vi "Generate Random GB of Size 2014-11-13.vi"() -> ()   [LabVIEW 2010]
uses:
  <vilib>/Utility/file.llb/Write To Spreadsheet File (string).vi
panel:
  out "# Created":i32
  out "Grain Boundary Definition":T1={"Grain 1 Orientation"=[1.0, 0.8858401549498205, 0.0], "Grain 2 Orientation"=[1.0, 0.3745791306245927, 0.0], "Twist Angle (Deg)"=39.42112887005932, "Translation Vector"=[0.0, 0.0, 0.0]}
  out "Current Index":i32=165102
  out "Status":string="Within range!\nNow creating...\nChecking expected size\nRolling dice...\n"
  in  "Make Random GBs Tab":T2(tab)=enum."Constraints"
  in  "Random Space":enum32{"Interface Plane", "Misorientation"}(tab)
  in  "Grain 1 Orientation":T3={"h, minimum"=1.0, "h, maximum"=1.0, "k, minimum"=0.0, "k, maximum"=1.0, "l, minimum"=0.0, "l, maximum"=1.0, "Force h>k>l ?"=TRUE} {"h, minimum" format="%#_4f"; "h, maximum" format="%#_4f"; "k, minimum" format="%#_4f"; "k, maximum" format="%#_4f"; "l, minimum" format="%#_4f"; "l, maximum" format="%#_4f"}
  in  "Random Translation?":bool
  in  "Twist Angle Max":dbl=64.0
  in  "Twist Angle Min":dbl
  in  "Grain 2 Orientation":T3={"h, minimum"=1.0, "h, maximum"=1.0, "k, minimum"=0.0, "k, maximum"=1.0, "l, minimum"=0.0, "l, maximum"=1.0, "Force h>k>l ?"=TRUE} {"h, minimum" format="%#_4f"; "h, maximum" format="%#_4f"; "k, minimum" format="%#_4f"; "k, maximum" format="%#_4f"; "l, minimum" format="%#_4f"; "l, maximum" format="%#_4f"}
  in  "Random Translation? Mis":bool
  in  "Mis Angle Max":dbl=64.0
  in  "Mis Angle Min":dbl
  in  "Misorientation Axis":T3={"h, minimum"=1.0, "h, maximum"=1.0, "k, minimum"=0.0, "k, maximum"=1.0, "l, minimum"=0.0, "l, maximum"=1.0, "Force h>k>l ?"=TRUE} {"h, minimum" format="%#_4f"; "h, maximum" format="%#_4f"; "k, minimum" format="%#_4f"; "k, maximum" format="%#_4f"; "l, minimum" format="%#_4f"; "l, maximum" format="%#_4f"}
  in  "Interface Plane from Grain 1":T3={"h, minimum"=1.0, "h, maximum"=1.0, "k, minimum"=0.0, "k, maximum"=1.0, "l, minimum"=0.0, "l, maximum"=1.0, "Force h>k>l ?"=TRUE} {"h, minimum" format="%#_4f"; "h, maximum" format="%#_4f"; "k, minimum" format="%#_4f"; "k, maximum" format="%#_4f"; "l, minimum" format="%#_4f"; "l, maximum" format="%#_4f"}
  in  "Nearest Integers?":bool
  in  "Max # of Atoms":i32=500
  in  "Require STEM Viewable?":bool
  in  "Grain Growth and Geometry":T4={"Grain 1 Length (prop)"=10.0, "Grain 2 Length (prop)"=10.0, "Max Grain Height (A)"=60.0, "Max Grain Width (A)"=60.0, "Grain 1 Start"=-0.001, "Overlap Region (A)"=0.001}
  in  "Min Seperation Distance (A)":dbl=2.0
  in  "Edge Duplication Range":dbl=3.0
  out "Expected # of atoms":i32=472
  out "# of atoms":i32=2541
  in  "Reduce to Repeating":T5={"Slab X"=4.6, "Slab Y"=4.0, "Tolerance (A)"=0.5, "Presorted?"=FALSE}
  in  "Output Directory":path=path "D:/Ab-initio/RAGB3"
  out "Last Creation Time":T6={"Time to create primitives"=1, "Time to Grow to Box"=5932, "Time to find subset"=6894, "Time to Cleanup"=0}
  out "Structures / Minute":dbl
  in  "Stop Making GBs":bool
  in  "Start Making GBs":bool
  in  "Making GBs":bool=TRUE
  in  "Conventional Unit Cell":T7={"Structure Name"="CdTe", "Lattice vector a"=[6.615785553057252, 0.0, 0.0], "Lattice vector b"=[0.0, 6.615785553057252, 0.0], "Lattice vector c"=[0.0, 0.0, 6.615785553057252], "Atoms Array"=[{"Atom Name"="Cd", "Positions (Direct)"=[[0.0, 0.0, 0.0], [0.0, 0.5, 0.5], [0.5, 0.0, 0.5], [0.5, 0.5, 0.0]], "Positions (Cartesian)"=[[0.0, 0.0, 0.0], [0.0, 3.307892776528626, 3.307892776528626], [3.307892776528626, 0.0, 3.307892776528626], [3.307892776528626, 3.307892776528626, 0.0]]}, {"Atom Name"="Te", "Positions (Direct)"=[[0.25, 0.25, 0.25], [0.75, 0.75, 0.25], [0.75, 0.25, 0.75], [0.25, 0.75, 0.75]], "Positions (Cartesian)"=[[1.653946388264313, 1.653946388264313, 1.653946388264313], [4.96183916479294, 4.96183916479294, 1.653946388264313], [4.96183916479294, 1.653946388264313, 4.96183916479294], [1.653946388264313, 4.96183916479294, 4.96183916479294]]}], "# of atoms"=8}
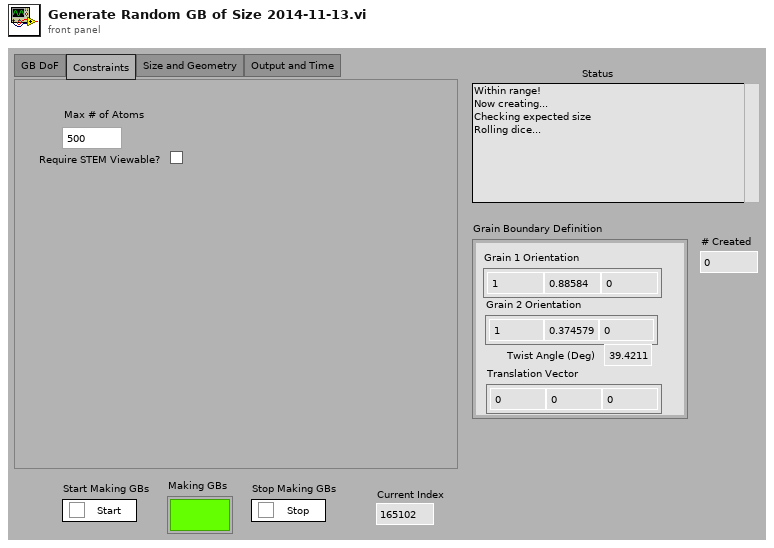
[diagram p1: front panel]
types:
  T1 = cluster{"Grain 1 Orientation":dbl[], "Grain 2 Orientation":dbl[], "Twist Angle (Deg)":dbl, "Translation Vector":dbl[]}
  T2 = enum32{"GB DoF", "Constraints", "Size and Geometry", "Output and Time"}
  T3 = cluster{"h, minimum":dbl, "h, maximum":dbl, "k, minimum":dbl, "k, maximum":dbl, "l, minimum":dbl, "l, maximum":dbl, "Force h>k>l ?":bool}
  T4 = cluster{"Grain 1 Length (prop)":dbl, "Grain 2 Length (prop)":dbl, "Max Grain Height (A)":dbl, "Max Grain Width (A)":dbl, "Grain 1 Start":dbl, "Overlap Region (A)":dbl}
  T5 = cluster{"Slab X":dbl, "Slab Y":dbl, "Tolerance (A)":dbl, "Presorted?":bool}
  T6 = cluster{"Time to create primitives":u32, "Time to Grow to Box":u32, "Time to find subset":u32, "Time to Cleanup":u32}
  T7 = cluster{"Structure Name":string, "Lattice vector a":dbl[], "Lattice vector b":dbl[], "Lattice vector c":dbl[], "Atoms Array":cluster{"Atom Name":string, "Positions (Direct)":dbl[][], "Positions (Cartesian)":dbl[][]}[], "# of atoms":i32}
  T8 = cluster{"Grain 1 Orientation":dbl[], "Grain 1 Orientation":dbl[], "Twist Angle (Deg)":dbl, "Translation Vector":dbl[]}
  T9 = cluster{"Grain 1 Orientation":dbl[], "Grain 2 Orientation":dbl[], "Twist Angle (Deg)":dbl}
  T10 = cluster{"Structure Name":string, "Lattice vector a":dbl[], "Lattice vector b":dbl[], "Lattice vector c":dbl[], "Atoms Array":cluster{"Atom Name":string, "Positions (Direct)":dbl[][], "Positions (Cartesian)":dbl[][]}[], "# of atoms":i32}[]
  T11 = typedef "NI_Matrix.lvlib/RealMatrix.ctl" = dbl[][]
  T12 = cluster{"Misorientation Angle":dbl, "Misorientation Axis, o":dbl[], "Misorientation Matrix":T11}
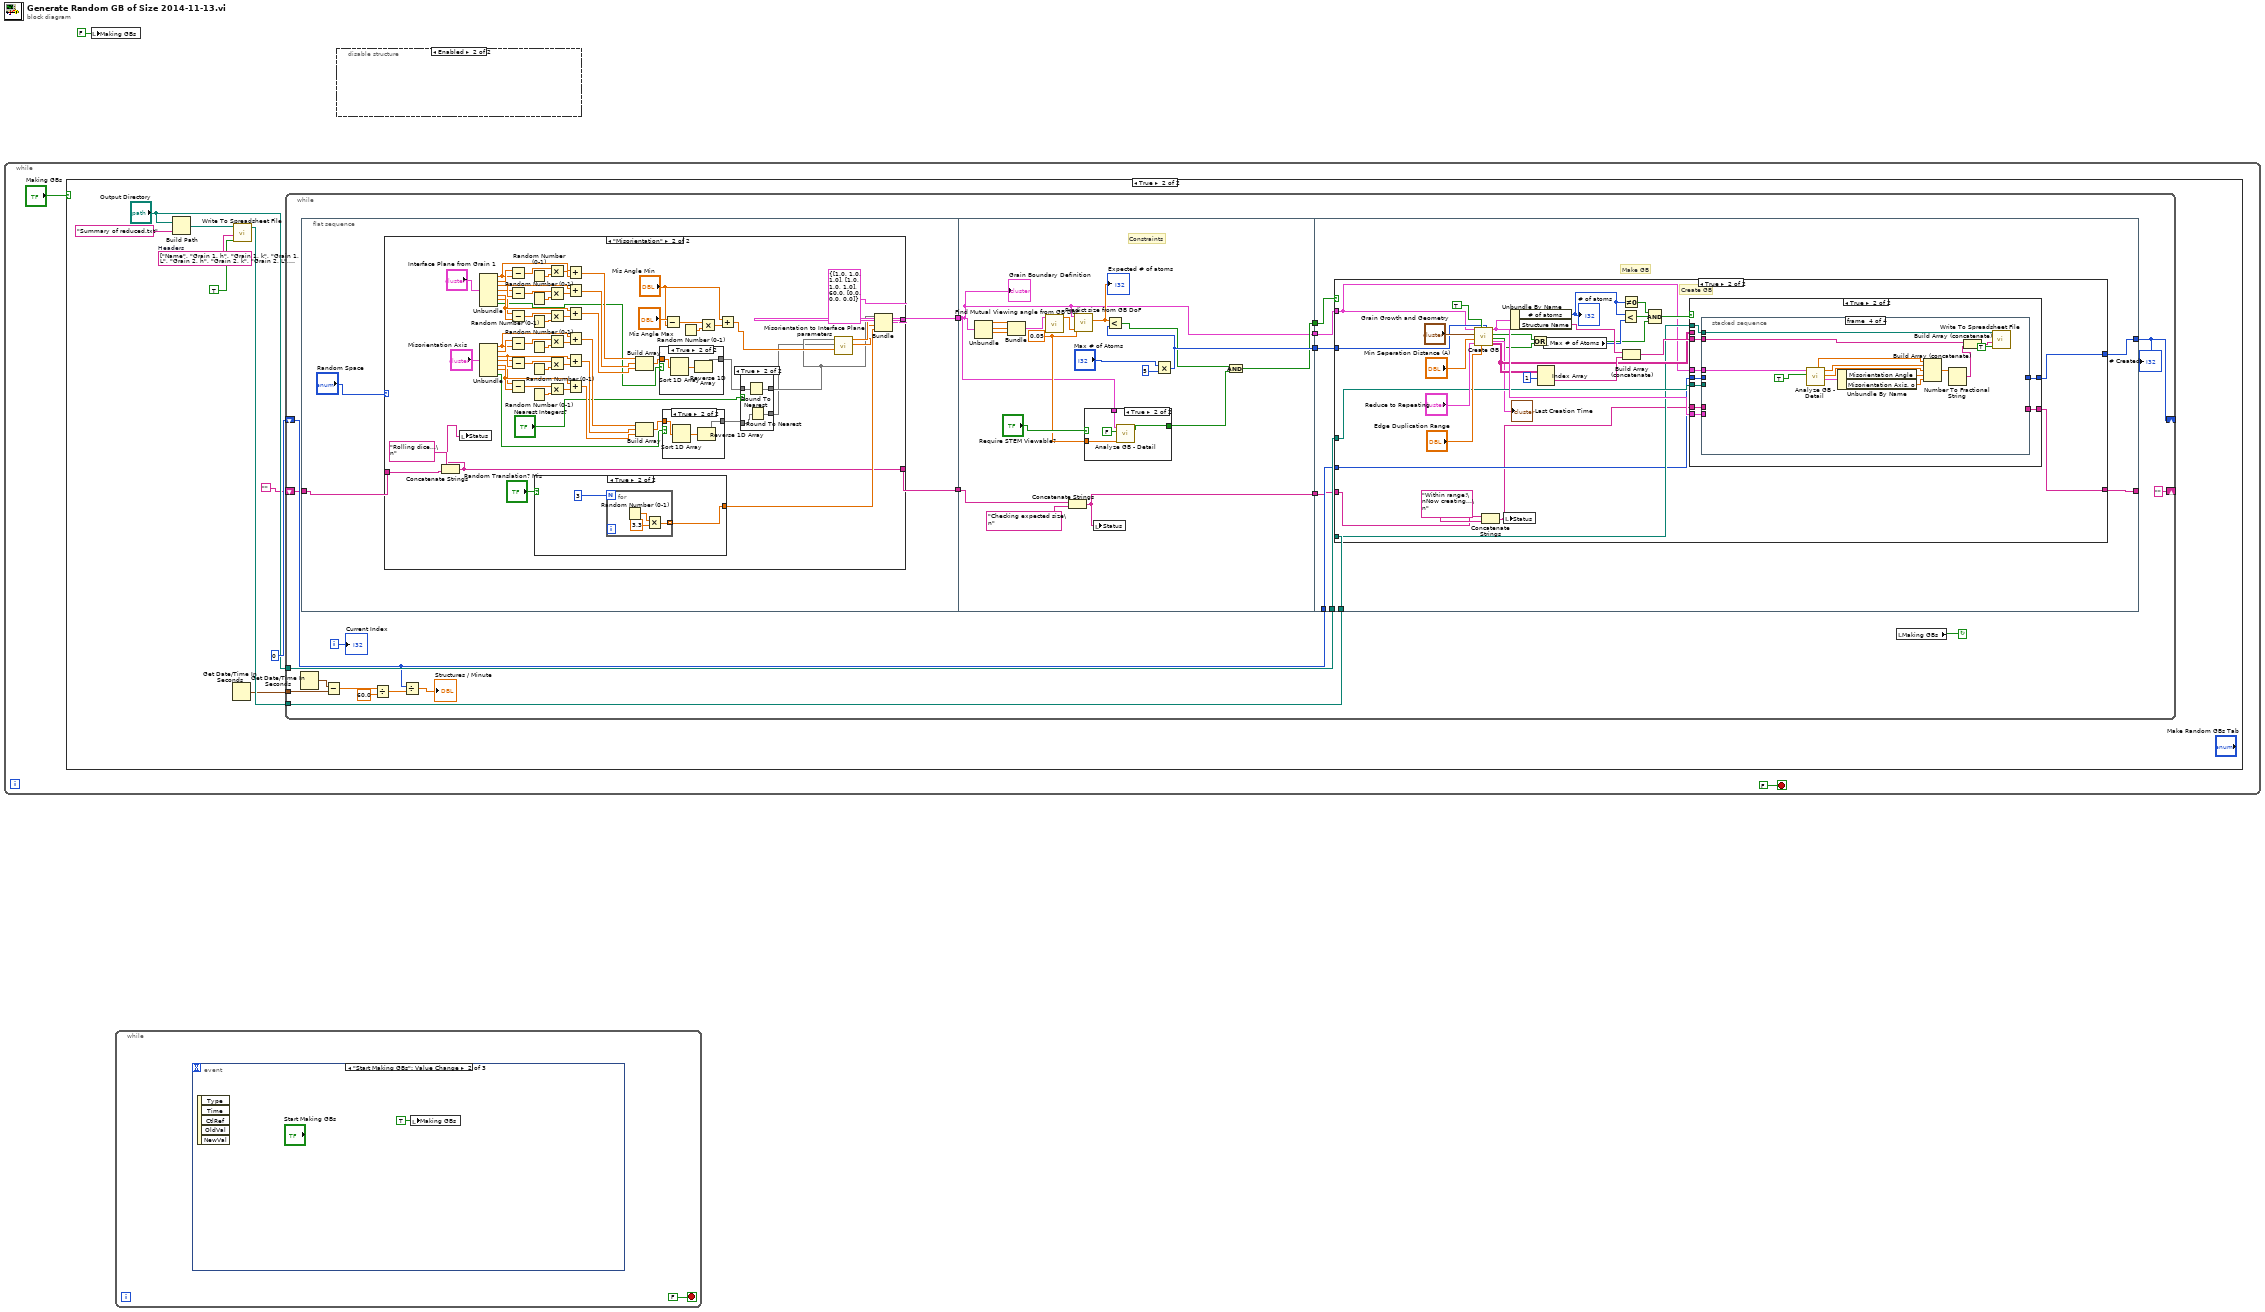
[diagram p0: block diagram]
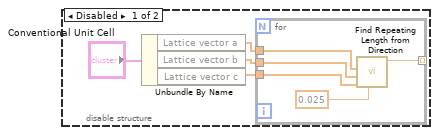
[diagram p2: hidden frame]
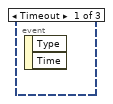
[diagram p3: hidden frame]
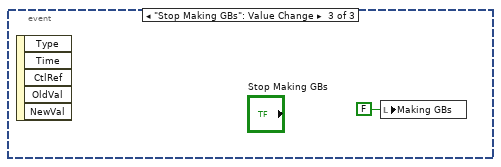
[diagram p4: hidden frame]
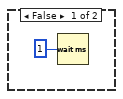
[diagram p5: hidden frame]
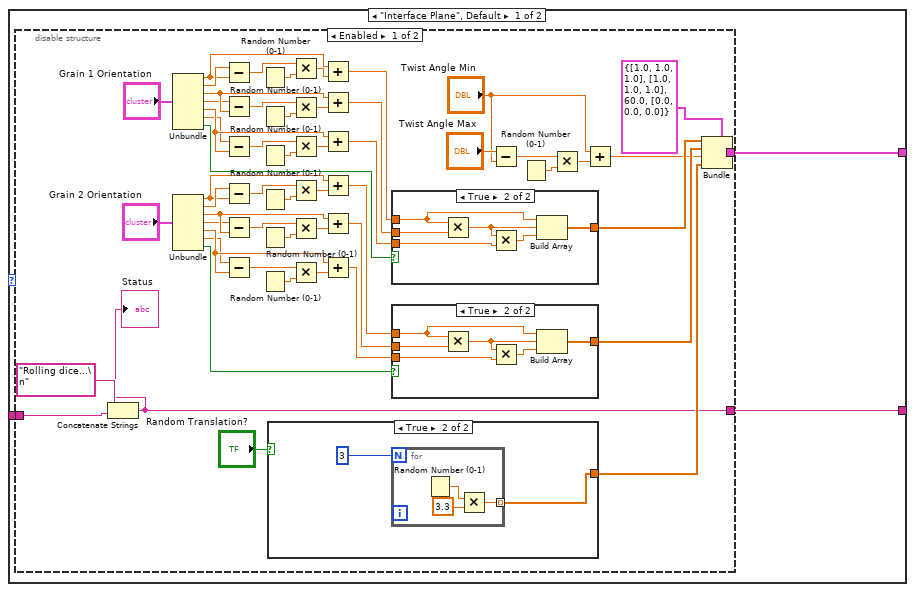
[diagram p6: hidden frame]
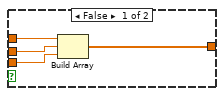
[diagram p7: hidden frame]
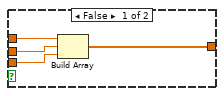
[diagram p8: hidden frame]
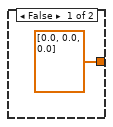
[diagram p9: hidden frame]
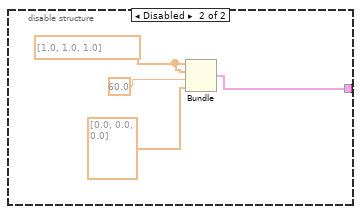
[diagram p10: hidden frame]
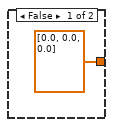
[diagram p14: hidden frame]
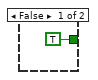
[diagram p15: hidden frame]
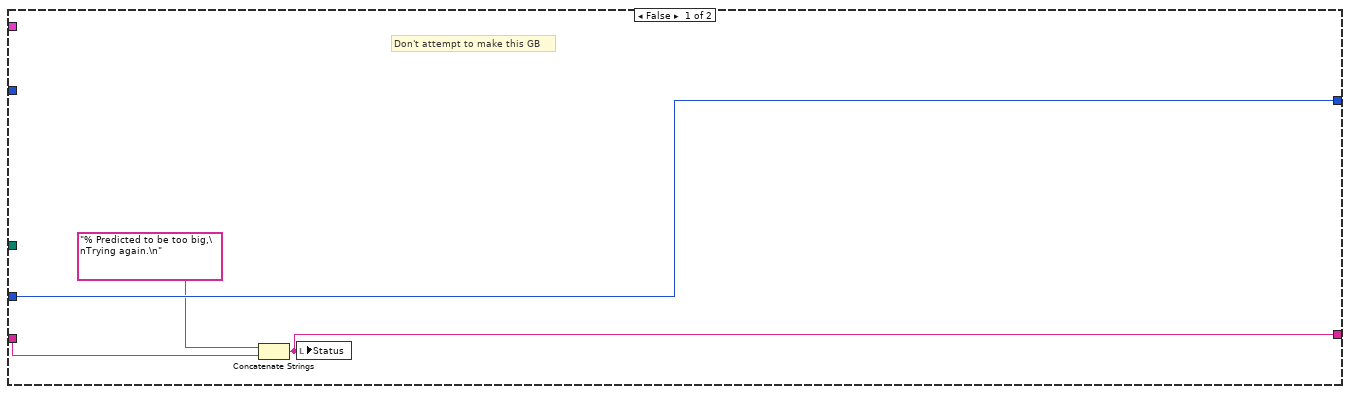
[diagram p16: hidden frame]
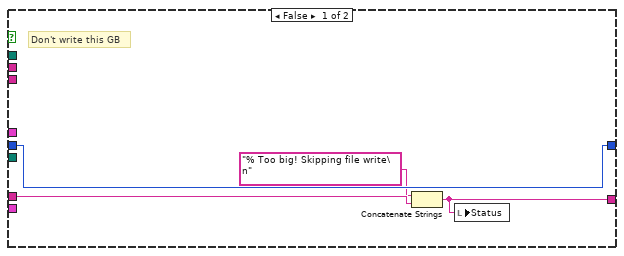
[diagram p17: hidden frame]
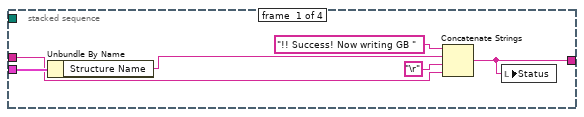
[diagram p18: hidden frame]
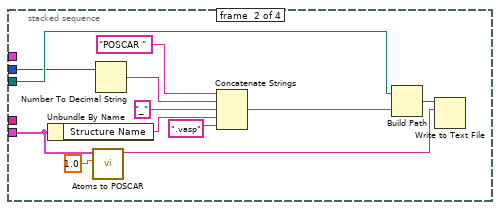
[diagram p19: hidden frame]
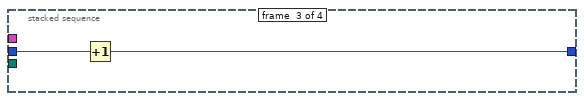
[diagram p20: hidden frame]
diagram:
  n1 = while {
    stop <- FALSE stop-if-true
    n2 = case shown="True" "Making GBs" {
      frame False {
        n3 = Wait (ms)(milliseconds to wait=u32 1) -> ()  [unwired: 1 out]
      }
      frame True {
        w9 = string[] ["Name", "Grain 1, h", "Grain 1, k", "Grain 1, L", "Grain 2, h", "Grain 2, k", "Grain 2, L", "Twist Angle (Deg)", "Translation Tx", "Translation Ty", "Translation Tz", "Tilt Angle (Deg)", "Viewing Angle, h", "Viewing Angle, k", "Viewing Angle, L", "Grain 1 Length (factor)", "Grain 2 Length (factor", "Max Grain Height (A)", "Max Grain Width (A)", "Grain 1 Start", "Overlap Region (A)", "Reduction Slab X", "Reduction Slab Y", "Reduction Tolerance (A)", "Min Atomic Separation Distance", "Edge Duplication Range", "# of Atoms", "STEM Direction,h", "STEM Direction,k", "STEM Direction,l", "Grain 1, [h]", "Grain 1, [k]", "Grain 1, [L]", "Grain 2, [h]", "Grain 2, [k]", "Grain 2, [L]", "Misorientaton Angle (Deg)", "Misorientation Axis, h", "Misorientation Axis, k", "Misorientation Axis, l"]  # Headers
        n4 = Build Path(base path="Output Directory", name or relative path="Summary of reduced.txt") -> (appended path=w10:path)
        n5 = Get Date/Time In Seconds() -> (seconds since 1Jan1904=w5:timestamp)
        n6 = call-poly <vilib>:"Write To Spreadsheet File.vi"("append to file? (new file:F)"=TRUE, "1D data"=w9, "file path (dialog if empty)"=w10) -> ("new file path (Not A Path if cancelled)"=w7:path)  [unwired: 5 in]
        n7 = while {
          shift-right: [w21] -> _
          shift-left: 0 -> [w22]
          tunnel: w5 -> [w29]
          tunnel: "Output Directory" -> [w24]
          tunnel: w7 -> [w23]
          shift-right: [""] -> _
          shift-left: "" -> [w20]
          i -> [w33]
          stop <- w17 continue-if-true
          n8 = Get Date/Time In Seconds() -> (seconds since 1Jan1904=w14:timestamp)
          n9 = flat-sequence {
            tunnel: [w37] -> w27
            tunnel: w20 -> [w36]
            tunnel: [w35] -> w19
            tunnel: w27 -> [w212]
            tunnel: [w212] -> w26
            tunnel: [w214] -> w25
            tunnel: w19 -> [w223]
            tunnel: [w221] -> w18
            tunnel: [w218] -> w15
            tunnel: w26 -> [w235]
            tunnel: w25 -> [w239]
            tunnel: w24 -> [w238]
            tunnel: w23 -> [w237]
            tunnel: w22 -> [w236]
            tunnel: [w234] -> w21
            tunnel: w18 -> [w233]
            tunnel: [w232] -> _
            tunnel: w15 -> [w231]
            frame #0 {
              n10 = case shown="\"Misorientation\"" "Random Space" {
                tunnel: [w40 w187] -> w37
                tunnel: w36 -> [w39 w140]
                tunnel: [w38 w135] -> w35
                frame "Interface Plane", Default {
                  n11 = disable-structure shown="Enabled" {
                    disable-tunnel: [w95 w122] -> w40
                    disable-tunnel: w39 -> [w43 _]
                    disable-tunnel: [w41 _] -> w38
                    frame Enabled {
                      n12 = Concatenate Strings(w43, "Rolling dice...\n" ("string")) -> (w41:string)
                      "Status" <- w41
                      n13 = Unbundle("Grain 1 Orientation") -> ("h, minimum"=w88:dbl, "h, maximum"=w91:dbl, "k, minimum"=w83:dbl, "k, maximum"=w82:dbl, "l, minimum"=w81:dbl, "l, maximum"=w80:dbl, "Force h>k>l ?"=w79:bool)
                      n14 = Unbundle("Grain 2 Orientation") -> ("h, minimum"=w68:dbl, "h, maximum"=w71:dbl, "k, minimum"=w63:dbl, "k, maximum"=w62:dbl, "l, minimum"=w61:dbl, "l, maximum"=w60:dbl, "Force h>k>l ?"=w59:bool)
                      n15 = Subtract(x=w91, y=w88) -> (x-y=w90:dbl)
                      n16 = Subtract(x=w82, y=w83) -> (x-y=w86:dbl)
                      n17 = Subtract(x=w80, y=w81) -> (x-y=w85:dbl)
                      n18 = Subtract(x=w71, y=w68) -> (x-y=w70:dbl)
                      n19 = Subtract(x=w62, y=w63) -> (x-y=w66:dbl)
                      n20 = Subtract(x=w60, y=w61) -> (x-y=w65:dbl)
                      n21 = Random Number (0-1)() -> (number: 0 to 1=w77:dbl)
                      n22 = Random Number (0-1)() -> (number: 0 to 1=w76:dbl)
                      n23 = Random Number (0-1)() -> (number: 0 to 1=w75:dbl)
                      n24 = Random Number (0-1)() -> (number: 0 to 1=w57:dbl)
                      n25 = Random Number (0-1)() -> (number: 0 to 1=w56:dbl)
                      n26 = Random Number (0-1)() -> (number: 0 to 1=w55:dbl)
                      n27 = case shown="True" "Random Translation?" {
                        tunnel: [dbl[] [0.0, 0.0, 0.0] w117] -> w94
                        frame False {
                        }
                        frame True {
                          n28 = for {
                            N: 3 -> [_]
                            tunnel: [w119] -> w117 mode=indexing
                            n29 = Random Number (0-1)() -> (number: 0 to 1=w121:dbl)
                            n30 = Multiply(x=w121, y=3.3) -> (x*y=w119:dbl)
                          }
                        }
                      }
                      n31 = Multiply(x=w90, y=w77) -> (x*y=w89:dbl)
                      n32 = Multiply(x=w86, y=w76) -> (x*y=w87:dbl)
                      n33 = Multiply(x=w85, y=w75) -> (x*y=w84:dbl)
                      n34 = Multiply(x=w70, y=w57) -> (x*y=w69:dbl)
                      n35 = Multiply(x=w66, y=w56) -> (x*y=w67:dbl)
                      n36 = Multiply(x=w65, y=w55) -> (x*y=w64:dbl)
                      n37 = Add(x=w88, y=w89) -> (x+y=w78:dbl)
                      n38 = Add(x=w83, y=w87) -> (x+y=w74:dbl)
                      n39 = Add(x=w81, y=w84) -> (x+y=w73:dbl)
                      n40 = Add(x=w68, y=w69) -> (x+y=w58:dbl)
                      n41 = Add(x=w63, y=w67) -> (x+y=w54:dbl)
                      n42 = Add(x=w61, y=w64) -> (x+y=w53:dbl)
                      n43 = case shown="True" w79 {
                        tunnel: w78 -> [w109 w113]
                        tunnel: w74 -> [w108 w115]
                        tunnel: w73 -> [w107 w114]
                        tunnel: [w106 w110] -> w72
                        frame False {
                          n44 = Build Array(w109, w108, w107) -> (w106:dbl[])
                        }
                        frame True {
                          n45 = Multiply(x=w113, y=w115) -> (x*y=w112:dbl)
                          n46 = Multiply(x=w112, y=w114) -> (x*y=w111:dbl)
                          n47 = Build Array(w113, w112, w111) -> (w110:dbl[])
                        }
                      }
                      n48 = case shown="True" w59 {
                        tunnel: w58 -> [w99 w103]
                        tunnel: w54 -> [w98 w105]
                        tunnel: w53 -> [w97 w104]
                        tunnel: [w96 w100] -> w52
                        frame False {
                          n49 = Build Array(w99, w98, w97) -> (w96:dbl[])
                        }
                        frame True {
                          n50 = Multiply(x=w103, y=w105) -> (x*y=w102:dbl)
                          n51 = Multiply(x=w102, y=w104) -> (x*y=w101:dbl)
                          n52 = Build Array(w103, w102, w101) -> (w100:dbl[])
                        }
                      }
                      n53 = Subtract(x="Twist Angle Max", y="Twist Angle Min") -> (x-y=w48:dbl)
                      n54 = Random Number (0-1)() -> (number: 0 to 1=w50:dbl)
                      n55 = Multiply(x=w48, y=w50) -> (x*y=w49:dbl)
                      n56 = Add(x="Twist Angle Min", y=w49) -> (x+y=w45:dbl)
                      n57 = Bundle(cluster=T1 {"Grain 1 Orientation"=[1.0, 1.0, 1.0], "Grain 2 Orientation"=[1.0, 1.0, 1.0], "Twist Angle (Deg)"=60.0, "Translation Vector"=[0.0, 0.0, 0.0]} ("Grain Boundary Definition"), "Grain 1 Orientation"=w72, "Grain 2 Orientation"=w52, "Twist Angle (Deg)"=w45, "Translation Vector"=w94) -> (w95:T1)
                    }
                    frame Disabled {
                      w125 = dbl[] [1.0, 1.0, 1.0] ("Grain 1 Orientation")
                      n58 = Bundle("Grain 1 Orientation"=w125, "Grain 1 Orientation"=w125, "Twist Angle (Deg)"=60.0, "Translation Vector"=dbl[] [0.0, 0.0, 0.0]) -> (w122:T8)  [unwired: 1 in]
                    }
                  }
                }
                frame "Misorientation" {
                  n59 = Concatenate Strings(w140, "Rolling dice...\n" ("string")) -> (w135:string)
                  n60 = local write "Status"(w135) -> ()
                  n61 = Unbundle("Interface Plane from Grain 1") -> ("h, minimum"=w180:dbl, "h, maximum"=w183:dbl, "k, minimum"=w175:dbl, "k, maximum"=w174:dbl, "l, minimum"=w173:dbl, "l, maximum"=w172:dbl, "Force h>k>l ?"=w129:bool)
                  n62 = Unbundle("Misorientation Axis") -> ("h, minimum"=w162:dbl, "h, maximum"=w165:dbl, "k, minimum"=w157:dbl, "k, maximum"=w156:dbl, "l, minimum"=w155:dbl, "l, maximum"=w154:dbl, "Force h>k>l ?"=w126:bool)
                  n63 = Subtract(x=w183, y=w180) -> (x-y=w182:dbl)
                  n64 = Subtract(x=w174, y=w175) -> (x-y=w178:dbl)
                  n65 = Subtract(x=w172, y=w173) -> (x-y=w177:dbl)
                  n66 = Subtract(x=w165, y=w162) -> (x-y=w164:dbl)
                  n67 = Subtract(x=w156, y=w157) -> (x-y=w160:dbl)
                  n68 = Subtract(x=w154, y=w155) -> (x-y=w159:dbl)
                  n69 = Random Number (0-1)() -> (number: 0 to 1=w170:dbl)
                  n70 = Random Number (0-1)() -> (number: 0 to 1=w169:dbl)
                  n71 = Random Number (0-1)() -> (number: 0 to 1=w168:dbl)
                  n72 = Random Number (0-1)() -> (number: 0 to 1=w152:dbl)
                  n73 = Random Number (0-1)() -> (number: 0 to 1=w151:dbl)
                  n74 = Random Number (0-1)() -> (number: 0 to 1=w150:dbl)
                  n75 = case shown="True" "Random Translation? Mis" {
                    tunnel: [dbl[] [0.0, 0.0, 0.0] w203] -> w186
                    frame False {
                    }
                    frame True {
                      n76 = for {
                        N: 3 -> [_]
                        tunnel: [w205] -> w203 mode=indexing
                        n77 = Random Number (0-1)() -> (number: 0 to 1=w207:dbl)
                        n78 = Multiply(x=w207, y=3.3) -> (x*y=w205:dbl)
                      }
                    }
                  }
                  n79 = Multiply(x=w182, y=w170) -> (x*y=w181:dbl)
                  n80 = Multiply(x=w178, y=w169) -> (x*y=w179:dbl)
                  n81 = Multiply(x=w177, y=w168) -> (x*y=w176:dbl)
                  n82 = Multiply(x=w164, y=w152) -> (x*y=w163:dbl)
                  n83 = Multiply(x=w160, y=w151) -> (x*y=w161:dbl)
                  n84 = Multiply(x=w159, y=w150) -> (x*y=w158:dbl)
                  n85 = Add(x=w180, y=w181) -> (x+y=w171:dbl)
                  n86 = Add(x=w175, y=w179) -> (x+y=w167:dbl)
                  n87 = Add(x=w173, y=w176) -> (x+y=w166:dbl)
                  n88 = Add(x=w162, y=w163) -> (x+y=w153:dbl)
                  n89 = Add(x=w157, y=w161) -> (x+y=w149:dbl)
                  n90 = Add(x=w155, y=w158) -> (x+y=w148:dbl)
                  n91 = Build Array(w171, w167, w166) -> (w130:dbl[])
                  n92 = Build Array(w153, w149, w148) -> (w128:dbl[])
                  n93 = case shown="True" w129 {
                    tunnel: [w192 w193] -> w131
                    tunnel: w130 -> [w192 w195]
                    frame False {
                    }
                    frame True {
                      n94 = Sort 1D Array(array=w195) -> (sorted array=w194:dbl[])
                      n95 = Reverse 1D Array(array=w194) -> (reversed array=w193:dbl[])
                    }
                  }
                  n96 = case shown="True" w126 {
                    tunnel: [w188 w189] -> w127
                    tunnel: w128 -> [w188 w190]
                    frame False {
                    }
                    frame True {
                      n97 = Sort 1D Array(array=w190) -> (sorted array=w191:dbl[])
                      n98 = Reverse 1D Array(array=w191) -> (reversed array=w189:dbl[])
                    }
                  }
                  n99 = Subtract(x="Mis Angle Max", y="Mis Angle Min") -> (x-y=w144:dbl)
                  n100 = Random Number (0-1)() -> (number: 0 to 1=w146:dbl)
                  n101 = Multiply(x=w144, y=w146) -> (x*y=w145:dbl)
                  n102 = Add(x="Mis Angle Min", y=w145) -> (x+y=w138:dbl)
                  n103 = case shown="True" "Nearest Integers?" {
                    tunnel: w127 -> [w196 w201]
                    tunnel: [w196 w200] -> w132
                    tunnel: w131 -> [w197 w199]
                    tunnel: [w197 w198] -> w133
                    frame False {
                    }
                    frame True {
                      n104 = Round To Nearest(number=w199) -> (nearest integer value=w198:dbl[])
                      n105 = Round To Nearest(number=w201) -> (nearest integer value=w200:dbl[])
                    }
                  }
                  n106 = call "Misorientation to Interface Plane parameters.vi"("Misorientation Angle"=w138, "Misorientation Axis, o"=w132, "Grain 1 Orientation"=w133) -> ("Twist Angle (Deg)"=w136:dbl, "Grain 2 Orientation"=w137:dbl[])  [unwired: 5 in, 2 out]
                  n107 = Bundle(cluster=T1 {"Grain 1 Orientation"=[1.0, 1.0, 1.0], "Grain 2 Orientation"=[1.0, 1.0, 1.0], "Twist Angle (Deg)"=60.0, "Translation Vector"=[0.0, 0.0, 0.0]} ("Grain Boundary Definition"), "Grain 1 Orientation"=w133, "Grain 2 Orientation"=w137, "Twist Angle (Deg)"=w136, "Translation Vector"=w186) -> (w187:T1)
                }
              }
            }
            frame #1 {
              w213 = 0.05 ("Integer Tolerance")
              # "Constraints"
              n108 = Unbundle(w212) -> ("Grain 1 Orientation"=w211:dbl[], "Grain 2 Orientation"=w210:dbl[], "Twist Angle (Deg)"=w209:dbl)  [unwired: 1 out]
              n109 = Bundle("Grain 1 Orientation"=w211, "Grain 2 Orientation"=w210, "Twist Angle (Deg)"=w209) -> (w208:T9)  [unwired: 1 in]
              n110 = call "Find Mutual Viewing angle from GB DoF.vi"("Grain Boundary Macro DoF"=w208) -> ("Mutual Viewing Angle"=w224:dbl[])  [unwired: 8 in, 2 out]
              n111 = Concatenate Strings(w223, "Checking expected size\n" ("string")) -> (w221:string)
              n112 = call "Predict size from GB DoF.vi"("Integer Tolerance"=w224, "Mutual Viewing Angle"=w213, "Grain Boundary Definition"=w212) -> ("Expected Volume (A3)"=w225:dbl)  [unwired: 6 in, 2 out]
              "Expected # of atoms" <- w225
              n113 = case shown="True" "Require STEM Viewable?" {
                tunnel: w212 -> [_ w229]
                tunnel: [TRUE ("STEM Viewable?") w228] -> w215
                tunnel: w213 -> [_ w227]
                frame False {
                }
                frame True {
                  n114 = call "Analyze GB - Detail.vi"("Integer Tolerance"=w227, "Find Integer Rep?"=FALSE, "Grain Boundary Definition"=w229) -> ("STEM Viewable?"=w228:bool)  [unwired: 1 in, 7 out]
                }
              }
              n115 = local write "Status"(w221) -> ()
              n116 = Multiply(x="Max # of Atoms", y=5) -> (x*y=w218:i32)
              n117 = Less?(x=w225, y=w218) -> (x < y?=w216:bool)
              n118 = And(x=w216, y=w215) -> (x .and. y?=w214:bool)
              "Grain Boundary Definition" <- w212
            }
            frame #2 {
              # "Make GB"
              n119 = case shown="True" w239 {
                tunnel: w238 -> [_ w263]
                tunnel: w237 -> [_ w262]
                tunnel: w236 -> [w243 w261]
                tunnel: w235 -> [_ w244]
                tunnel: [w243 w253] -> w234
                tunnel: w233 -> [w242 w251]
                tunnel: [w240 w249] -> w232
                tunnel: w231 -> [_ w245]
                frame False {
                  # "Don't attempt to make this GB"
                  n120 = Concatenate Strings("% Predicted to be too big,\nTrying again.\n" ("string"), w242) -> (w240:string)
                  n121 = local write "Status"(w240) -> ()
                }
                frame True {
                  # "Create GB"
                  n122 = call "Create GB.vi"("Max # of atoms"=w245, "Edge Duplication Range"="Edge Duplication Range", "Skip cleanup if no subset"=TRUE, "Reduce to Repeating"="Reduce to Repeating", "Min Seperation Distance (A)"="Min Seperation Distance (A)", "Grain Growth and Geometry"="Grain Growth and Geometry", "Grain Boundary Definition"=w244) -> ("GB Data"=w268:string[][], "Reduced Orthorhombic?"=w247:bool, "Reduced Rhombahedral?"=w248:bool, "Grain Boundary"=w269:T7, "Ortho and Rhom"=→"Last Creation Time":T10)
                  n123 = Concatenate Strings(w251, "Within range!\nNow creating...\n" ("string")) -> (w250:string)
                  n124 = local write "Status"(w250) -> ()
                  n125 = Unbundle By Name(w269) -> ("# of atoms"=w257:i32, "Structure Name"=w273:string)
                  "# of atoms" <- w257
                  n126 = Or(x=w248, y=w247) -> (x .or. y?=w246:bool)
                  n127 = Index Array(array=w268, index (row)=1) -> (element=w271:string[])  [unwired: 1 in]
                  n128 = local read "Max # of Atoms"() -> (w258:i32)
                  n129 = Less?(x=w257, y=w258) -> (x < y?=w255:bool)
                  n130 = Not Equal To 0?(x=w257) -> (x != 0?=w256:bool)
                  n131 = Build Array (concatenate)(w273, w271) -> (w272:string[])
                  n132 = Compound Arithmetic op=AND(w256, w255, w246) -> (w254:bool)
                  n133 = case shown="True" w254 {
                    tunnel: w261 -> [w277 w284]
                    tunnel: [w277 w283] -> w253
                    tunnel: w268 -> [_ _]
                    tunnel: w269 -> [_ w286]
                    tunnel: w272 -> [_ w281]
                    tunnel: w263 -> [_ w285]
                    tunnel: w262 -> [_ w282]
                    tunnel: w250 -> [w276 w279]
                    tunnel: [w275 w278] -> w249
                    tunnel: w244 -> [_ w280]
                    frame False {
                      # "Don't write this GB"
                      n134 = Concatenate Strings("% Too big! Skipping file write\n" ("string"), w276) -> (w275:string)
                      n135 = local write "Status"(w275) -> ()
                    }
                    frame True {
                      n136 = stacked-sequence {
                        tunnel: w286 -> [w290 w304 _ _]
                        tunnel: w285 -> [_ w299 _ _]
                        tunnel: w284 -> [_ w297 w306 _]
                        tunnel: [_ _ w305 _] -> w283
                        tunnel: w282 -> [_ _ _ w320]
                        tunnel: w281 -> [_ _ _ w318]
                        tunnel: w280 -> [_ _ _ w312]
                        tunnel: w279 -> [w288 _ _ _]
                        tunnel: [w287 _ _ _] -> w278
                        frame #0 {
                          n137 = Unbundle By Name(w290) -> ("Structure Name"=w289:string)
                          n138 = Concatenate Strings("!! Success! Now writing GB " ("string"), w289, "\r", w288) -> (w287:string)
                          n139 = local write "Status"(w287) -> ()
                        }
                        frame #1 {
                          n140 = Unbundle By Name(w304) -> ("Structure Name"=w294:string)
                          n141 = call "Atoms to POSCAR.vi"("Volume Factor"=1.0, "Atomic Structure"=w304) -> ("POSCAR File"=w296:string)  [unwired: 9 in]
                          n142 = Number To Decimal String(number=w297) -> (decimal integer string=w303:string)  [unwired: 1 in]
                          n143 = Concatenate Strings("POSCAR " ("string"), w303, "_" ("string"), w294, ".vasp" ("string")) -> (w302:string)
                          n144 = Build Path(base path=w299, name or relative path=w302) -> (appended path=w301:path)
                          n145 = Write to Text File(file (use dialog)=w301, text=w296) -> ()  [unwired: 2 in, 3 out]
                        }
                        frame #2 {
                          n146 = Increment(x=w306) -> (x+1=w305:i32)
                        }
                        frame #3 {
                          n147 = call "Analyze GB - Detail.vi"("Find Integer Rep?"=TRUE, "Grain Boundary Definition"=w312) -> ("Misorientation"=w316:T12, "Grain 2 Integers"=w315:dbl[], "Grain 1 Integers"=w314:dbl[], "Suggested view direction"=w307:dbl[])  [unwired: 2 in, 4 out]
                          n148 = Unbundle By Name(w316) -> ("Misorientation Angle"=w311:dbl, "Misorientation Axis, o"=w310:dbl[])
                          n149 = Build Array (concatenate)(w307, w314, w315, w311, w310) -> (w309:dbl[])
                          n150 = Number To Fractional String(number=w309) -> (F-format string=w308:string[])  [unwired: 3 in]
                          n151 = Build Array (concatenate)(w318, w308) -> (w317:string[])
                          n152 = call-poly <vilib>:"Write To Spreadsheet File.vi"("append to file? (new file:F)"=TRUE, "1D data"=w317, "file path (dialog if empty)"=w320) -> ()  [unwired: 5 in, 1 out]
                        }
                      }
                    }
                  }
                }
              }
            }
          }
          n153 = Subtract(x=w14, y=w29) -> (x-y=w31:dbl)
          n154 = Divide(x=w31, y=60.0) -> (x/y=w28:dbl)
          n155 = Divide(x=w22, y=w28) -> (x/y=→"Structures / Minute":dbl)
          n156 = local read "Making GBs"() -> (w17:bool)
          "Current Index" <- w33
          "# Created" <- w21
        }
      }
    }
  }
  n157 = local write "Making GBs"(FALSE ("Making GBs")) -> ()
  n158 = while {
    stop <- FALSE stop-if-true
    n159 = event shown="[1] \"Start Making GBs\": Value Change" {
      selector: _ -> [_ _ _]
      dyn-events: _ -> [_ _ _]
      timeout: _ -> [_ _ _]
      event Timeout {
        n160 = event-data() -> ()  [unwired: 1 in, 2 out]
      }
      event "Start Making GBs": Value Change {
        n161 = event-data() -> ()  [unwired: 1 in, 5 out]
        n162 = local write "Making GBs"(TRUE ("Making GBs")) -> ()
      }
      event "Stop Making GBs": Value Change {
        n163 = event-data() -> ()  [unwired: 1 in, 5 out]
        n164 = local write "Making GBs"(FALSE ("Making GBs")) -> ()
      }
    }
  }
  n165 = disable-structure shown="Enabled" {
    frame Disabled {
      n166 = Unbundle By Name("Conventional Unit Cell") -> ("Lattice vector a"=w325:dbl[], "Lattice vector b"=w326:dbl[], "Lattice vector c"=w327:dbl[])
      n167 = for {
        tunnel: w325 -> [w332]
        tunnel: w326 -> [w331]
        tunnel: w327 -> [w330]
        tunnel: [w328] -> _ mode=indexing
        n168 = call "Find Repeating Length from Direction.vi"("Tolerance"=0.025, "Lattice vector c"=w330, "Lattice vector b"=w331, "Lattice vector a"=w332) -> ("Repeating Length (A)"=w328:dbl)  [unwired: 7 in]
      }
    }
    frame Enabled {
    }
  }
